vi "Test_InverseLogic_WriteZero_TerminalVisible.vi"(8 "error in (no error)":errorcluster, 11 "TestCase in":refnum<class "TestTerminalVisibilityBinding.lvclass">) -> (0 "error out":errorcluster, 3 "TestCase out":refnum<class "TestTerminalVisibilityBinding.lvclass">)   [LabVIEW 2017, in "TestTerminalVisibilityBinding.lvclass"]
uses:
  TestTerminalVisibilityBinding.lvclass
  Source/Concrete/TerminalVisibilityBinding/TerminalVisibilityBinding.lvclass
  C:/Git/composed-transport/Source/ITransport/ITransport.lvclass
  Source/ITransport/ITransport.lvclass
panel:
  in  "Numeric":i32
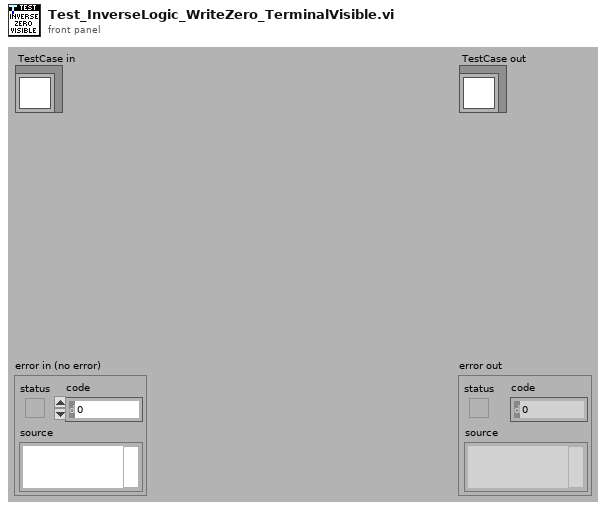
[diagram p1: front panel]
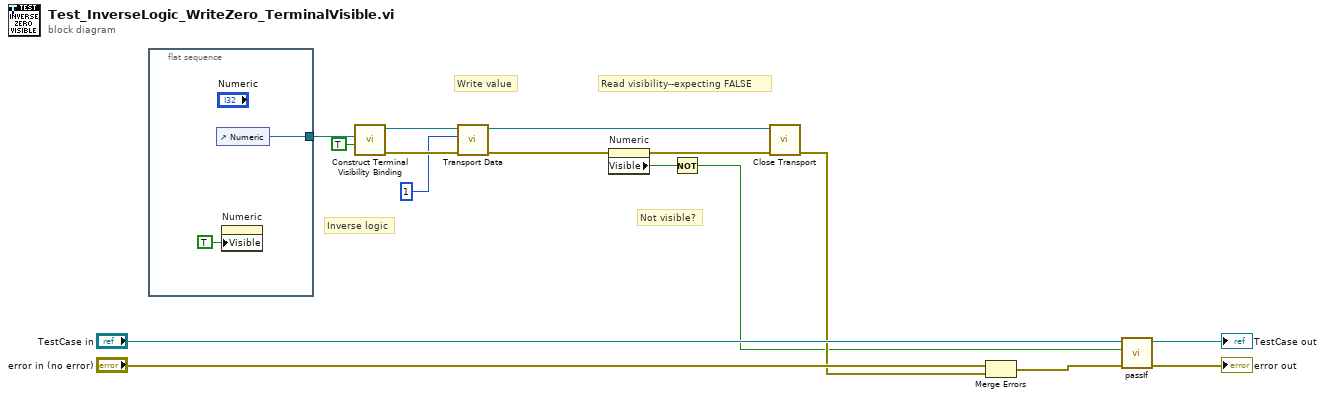
[diagram p0: block diagram]
diagram:
  # "Not visible?"
  # "Inverse logic"
  # "Read visibility--expecting FALSE"
  # "Write value"
  n1 = flat-sequence {
    tunnel: [w18] -> w7
    frame #0 {
      n2 = control-ref of="Numeric"() -> (w18:refnum<vi>)
      n3 = property on="Numeric" class="DigNum (strict)"("Visible"=TRUE) -> ()  [unwired: 2 in, 2 out]
    }
  }
  n4 = call "Construct Terminal Visibility Binding.vi"("Inverse Visible Logic? (F)"=TRUE, "Ctl Refnum"=w7) -> ("error out"=w10:errorcluster, "TerminalVisibilityBinding"=w12:refnum<class "TerminalVisibilityBinding.lvclass">)  [unwired: 8 in]
  n5 = call "Transport Data.vi"("error in (no error)"=w10, "Value"=1, "ITransport in"=w12) -> ("error out"=w6:errorcluster, "ITransport out"=w8:refnum<class "TerminalVisibilityBinding.lvclass">)  [unwired: 7 in]
  n6 = property on="Numeric" class="DigNum (strict)"(error in=w6) -> (error out=w5:errorcluster, "Visible"=w4:bool)  [unwired: 1 in, 1 out]
  n7 = Not(x=w4) -> (.not. x?=w1:bool)
  n8 = call-dynamic "Close Transport.vi"("error in (no error)"=w5, "ITransport in"=w8) -> ("error out"=w3:errorcluster)  [unwired: 9 in]
  n9 = Merge Errors("error in (no error)", w3) -> (w11:errorcluster)
  n10 = call-dynamic "passIf.vi"("error in (no error)"=w11, "pass"=w1, "TestCase in"="TestCase in") -> ("error out"=→"error out":errorcluster, "TestCase out"=→"TestCase out":refnum<class "TestTerminalVisibilityBinding.lvclass">)  [unwired: 7 in]
